vi "Robot Constants.vi"() -> (3 "Robot Data":T1)   [LabVIEW 2020]
uses:
  <vilib>/Rock Robotics/Network Tables/NT Read Number.vi
panel:
  in  "Shooter Table":dbl[][](array[numeric])=[[8.0, 0.0, 6.0, 0.0], [4900.0, 3100.0, 4850.0, 0.0], [0.8, 0.7, 0.63, 0.0]]
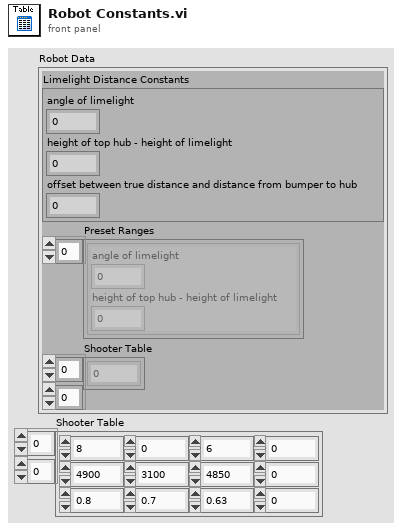
[diagram p1: front panel]
types:
  T1 = cluster{"Limelight Distance Constants":cluster{"angle of limelight":dbl, "height of top hub - height of limelight":dbl, "offset between true distance and distance from bumper to hub":dbl}, "Preset Ranges":cluster{"angle of limelight":dbl, "height of top hub - height of limelight":dbl}[], "Shooter Table":dbl[][]}
  T2 = cluster{"angle of limelight":dbl, "height of top hub - height of limelight":dbl, "offset between true distance and distance from bumper to hub":dbl}
  T3 = cluster{"angle of limelight":dbl, "height of top hub - height of limelight":dbl}[]
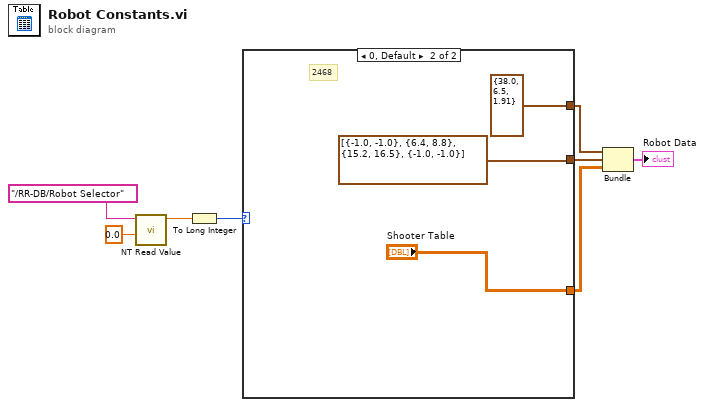
[diagram p0: block diagram]
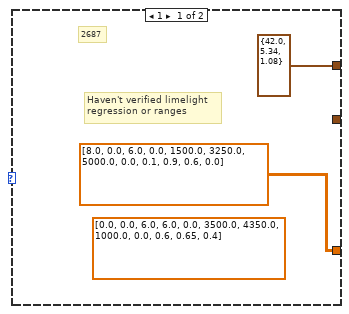
[diagram p2: hidden frame]
diagram:
  n1 = call-poly <vilib>:"NT Read Value.vi"("Default Value"=0.0, "Name"="/RR-DB/Robot Selector") -> ("Numeric"=w7:dbl)  [unwired: 8 in, 1 out]
  n2 = To Long Integer(number=w7) -> (32bit integer=w6:i32)
  n3 = case shown="0, Default" w6 {
    tunnel: [T2 {"angle of limelight"=42.0, "height of top hub - height of limelight"=5.34, "offset between true distance and distance from bumper to hub"=1.08} ("Limelight Distance Constants") T2 {"angle of limelight"=38.0, "height of top hub - height of limelight"=6.5, "offset between true distance and distance from bumper to hub"=1.91} ("Limelight Distance Constants")] -> w4
    tunnel: [dbl[][] [[8.0, 0.0, 6.0, 0.0], [1500.0, 3250.0, 5000.0, 0.0], [0.1, 0.9, 0.6, 0.0]] ("Shooter Table") "Shooter Table"] -> w3
    tunnel: [_ T3 [{"angle of limelight"=-1.0, "height of top hub - height of limelight"=-1.0}, {"angle of limelight"=6.4, "height of top hub - height of limelight"=8.8}, {"angle of limelight"=15.2, "height of top hub - height of limelight"=16.5}, {"angle of limelight"=-1.0, "height of top hub - height of limelight"=-1.0}] ("Preset Ranges")] -> w2
    frame 1 {
      (unwired) dbl[][] [[0.0, 0.0, 6.0, 6.0], [0.0, 3500.0, 4350.0, 1000.0], [0.0, 0.6, 0.65, 0.4]] ("Shooter Table")
      # "Haven't verified limelight\nregression or ranges"
      # "2687"
    }
    frame 0, Default {
      # "2468"
    }
  }
  n4 = Bundle("Limelight Distance Constants"=w4, "Preset Ranges"=w2, "Shooter Table"=w3) -> (→"Robot Data":T1)  [unwired: 1 in]
